vi "InitializeSessions.vi"(0 "Keysight_34401A-DMM in":refnum<class "Keysight_34401A-DMM.lvclass">, 5 "InitializeSessionsInfo":variant, 11 "error in (no error)":errorcluster) -> (4 "Keysight_34401A-DMM out":refnum<class "Keysight_34401A-DMM.lvclass">, 15 "error out":errorcluster)   [LabVIEW 2020, in "AbstractDMM.lvlib" / "Keysight_34401A-DMM.lvclass"]
uses:
  Keysight_34401A-DMM.lvclass
  TypeDef/Initialize_Information.ctl
  <vilib>/MeasurementLink/MeasurementLink Session Management V1/Session Reservation/Initialize and Close Session Behavior.ctl
  Keysight_34401A-DMM.lvclass/Keysight_34401A-DMM.ctl
  Base/AbstractDMM.lvclass
  Keysight 34401A DMM Instrument.lvlib
  <vilib>/MeasurementLink/MeasurementLink Session Management V1/Session Reservation/Session Reservation.lvclass
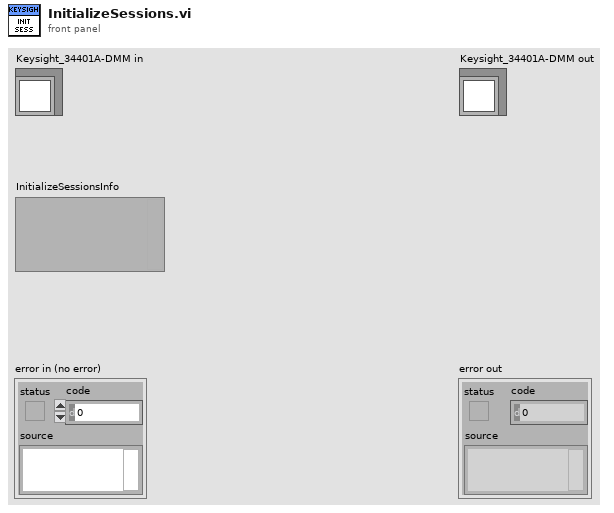
[diagram p1: front panel]
types:
  T1 = cluster{"Baud Rate":u32, "Parity":u16, "Data Bits":u16}
  T2 = typedef "AbstractDMM.lvlib/Keysight_34401A-DMM.lvclass/Initialize_Information.ctl" = cluster{"initialize and close session behavior":T3, "reset":bool}
  T3 = typedef "MeasurementLink Session Management V1.lvlib/Session Reservation.lvclass/Initialize and Close Session Behavior.ctl" = enum16{"Auto", "Initialize and Close", "Attach and Detach", "Initialize and Detach", "Attach and Close"}
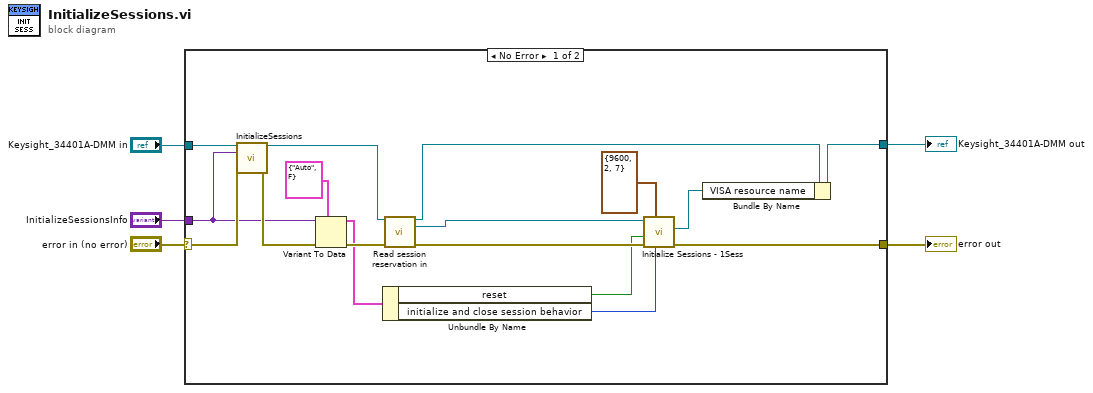
[diagram p0: block diagram]
diagram:
  n1 = case shown="No Error" "error in (no error)" {
    selector: "error in (no error)" -> [w21 w23]
    tunnel: "Keysight_34401A-DMM in" -> [w22 w24]
    tunnel: [w17 w23] -> w3
    tunnel: "InitializeSessionsInfo" -> [w14 _]
    tunnel: [w8 w24] -> w1
    frame No Error {
      n2 = call-parent "InitializeSessions.vi"("AbstractDMM in"=w22, "InitializeSessionsInfo"=w14, "error in (no error)"=w21) -> ("AbstractDMM out"=w20:refnum<class "Keysight_34401A-DMM.lvclass">, "error out"=w19:errorcluster)  [unwired: 11 in]
      n3 = Variant To Data(error in=w19, type=T2 {"initialize and close session behavior"=enum."Auto", "reset"=FALSE} ("Initialize_Information"), Variant=w14) -> (data=w12:T2, error out=w15:errorcluster)
      n4 = Unbundle By Name(w12) -> ("reset"=w10:bool, "initialize and close session behavior"=w11:T3)
      n5 = call-dynamic "Read session reservation in.vi"("AbstractDMM in"=w20, "error in (no error)"=w15) -> ("AbstractDMM out"=w13:refnum<class "Keysight_34401A-DMM.lvclass">, "MeasurementLink Session Management V1.lvlib:Session Reservation.lvclass"=w16:refnum<class "Session Reservation.lvclass">, "error out"=w18:errorcluster)  [unwired: 11 in]
      n6 = call "Initialize Sessions - 1Sess.vi"("initialize and close session behavior"=w11, "serial configuration"=T1 {"Baud Rate"=9600, "Parity"=2, "Data Bits"=7}, "error in"=w18, "reset"=w10, "session reservation in"=w16) -> ("error out"=w17:errorcluster, "session"=w7:refnum<visa-resource-name>)  [unwired: 3 in, 2 out]
      n7 = Bundle By Name(cluster=w13, "VISA resource name"=w7) -> (w8:refnum<class "Keysight_34401A-DMM.lvclass">)
    }
    frame Error {
    }
  }
  "error out" <- w3
  "Keysight_34401A-DMM out" <- w1
